vi "OA_Col-Setting.vi"(0 "Origin.Column":refnum<k7>, 1 "Type":i32(ring)=-1 items=["COLTYPE_NO_CHANGE"=-1, "COLTYPE_Y"=0, "COLTYPE_NONE"=1, "COLTYPE_ERROR"=2, "COLTYPE_X"=3, "COLTYPE_LABEL"=4, "COLTYPE_Z"=5, "COLTYPE_X_ERROR"=6, "COLTYPE_GROUP"=7, "COLTYPE_SUBJECT"=8], 2 "LongName":string, 3 "Units":string, 4 "error in (no error)":errorcluster, 5 "DataFormat":i32(ring)=-1 items=["DF_NO_CHANGE"=-1, "DF_DOUBLE"=0, "DF_TEXT"=1, "DF_TIME"=2, "DF_DATE"=3, "DF_TEXT_NUMERIC"=9, "DF_FLOAT"=32, "DF_SHORT"=33, "DF_LONG"=34, "DF_CHAR"=35, "DF_BYTE"=38, "DF_USHORT"=39, "DF_ULONG"=40, "DF_COMPLEX"=41], 7 "Comments":string) -> (6 "Origin.Column Out":refnum<k7>, 8 "error out":errorcluster)   [LabVIEW 2010]
doc: "Set various Column properties\n\nType:\n Column designation, X, Y etc, default is not to make any changes\nDataFormat:\n Internal array data type, like array of double, complex etc. \n Default is not to change\nLongName, Units, Comments:\n Column labels, default will clear them, so you must supply the string\n if you don't want these labels reset to empty."
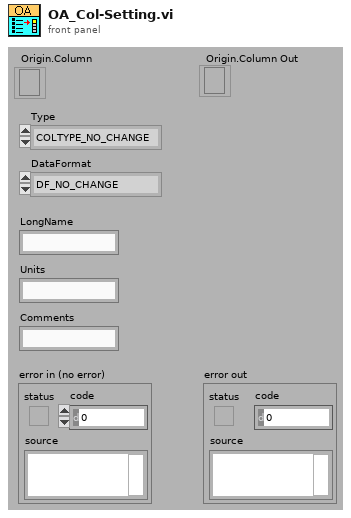
[diagram p1: front panel]
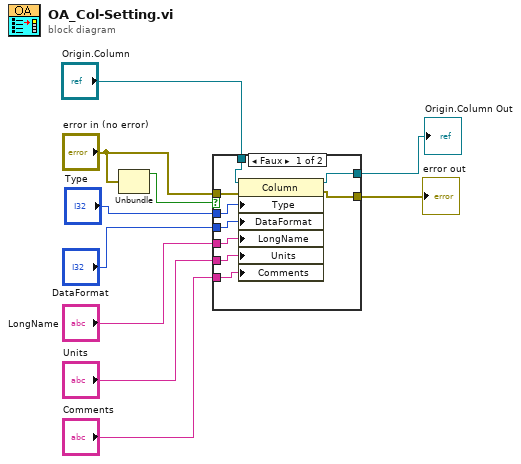
[diagram p0: block diagram]
diagram:
  n1 = Unbundle("error in (no error)") -> ("status"=w5:bool)  [unwired: 2 out]
  n2 = case shown="Faux" w5 {
    tunnel: "error in (no error)" -> [w19 w21]
    tunnel: "LongName" -> [w17 _]
    tunnel: "Units" -> [w16 _]
    tunnel: "Comments" -> [w15 _]
    tunnel: [w14 w21] -> w7
    tunnel: "Origin.Column" -> [w18 w20]
    tunnel: [w13 w20] -> w3
    tunnel: "Type" -> [w12 _]
    tunnel: "DataFormat" -> [w11 _]
    frame False {
      n3 = property class="Column"(reference=w18, error in=w19, "Type"=w12, "DataFormat"=w11, "LongName"=w17, "Units"=w16, "Comments"=w15) -> (reference out=w13:refnum<k7>, error out=w14:errorcluster)
    }
    frame True {
    }
  }
  "error out" <- w7
  "Origin.Column Out" <- w3
